vi "How to use in host.vi"(11 "Select Part":u16(ring) items=["P1.jpg", "P10.JPG", "P11.JPG", "P12.JPG", "P13.JPG", "P14.JPG", "P2.JPG", "P3.JPG", "P4.JPG", "P5.JPG", "P6.JPG", "P7.JPG", "P8.JPG", "P9.JPG"]) -> (1 "2D Picture":picture)   [LabVIEW 2015]
panel:
  out "error out":errorcluster
  out "empty?":bool
  in  "stop":bool
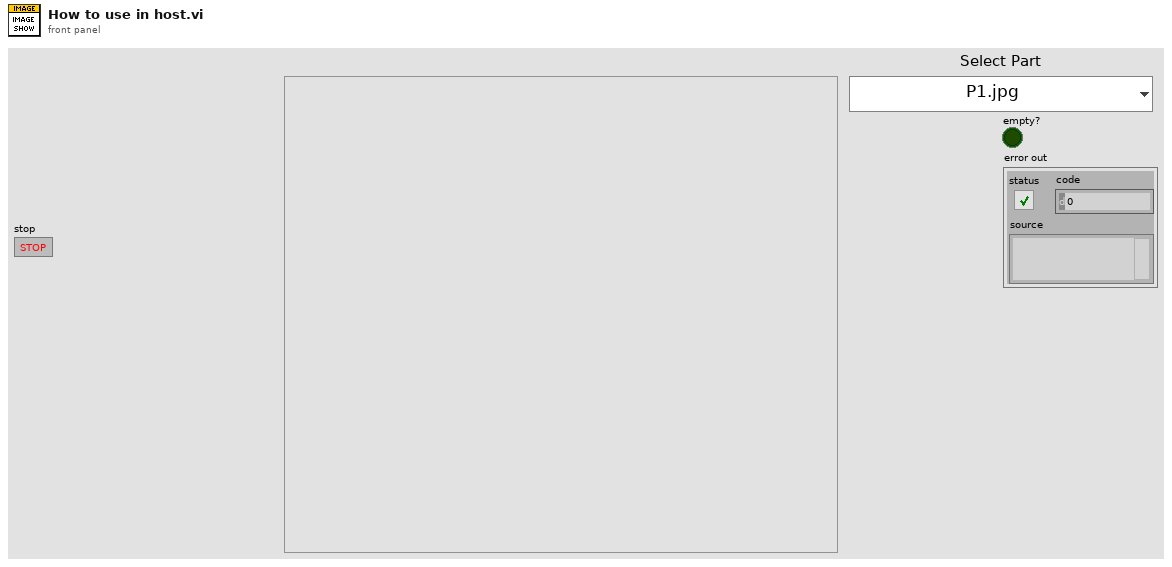
[diagram p1: front panel]
types:
  T1 = typedef "imagedata.ctl" = cluster{"image type":i32, "image depth":i32, "image":u8[], "mask":u8[], "colors":u32[], "Rectangle":cluster{"left":i16, "top":i16, "right":i16, "bottom":i16}}
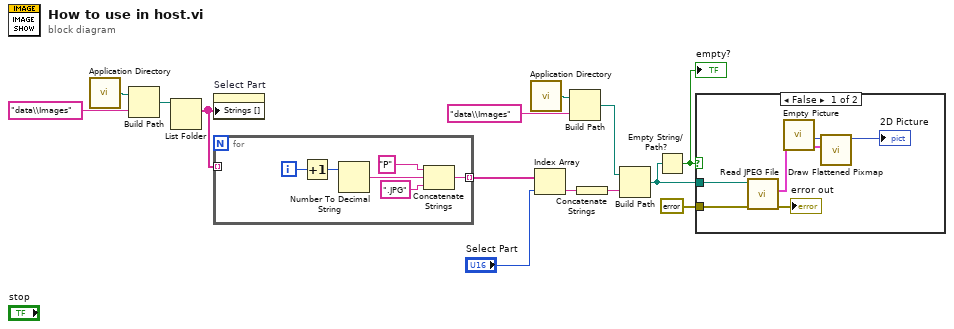
[diagram p0: block diagram]
diagram:
  n1 = call <vilib>:"Application Directory.vi"() -> ("Application Directory"=w14:path)
  n2 = Build Path(base path=w14, name or relative path="data\\Images") -> (appended path=w12:path)
  n3 = List Folder(path=w12) -> (filenames=w2:string[])  [unwired: 3 in, 3 out]
  n4 = property on="Select Part" class="Ring (strict)"("Strings []"=w2) -> ()  [unwired: 2 in, 2 out]
  n5 = for {
    tunnel: w2 -> [_] mode=indexing
    tunnel: [w15] -> w1 mode=indexing
    i -> [w19]
    n6 = Increment(x=w19) -> (x+1=w17:i32)
    n7 = Number To Decimal String(number=w17) -> (decimal integer string=w18:string)  [unwired: 1 in]
    n8 = Concatenate Strings("P" ("string"), w18, ".JPG" ("string")) -> (w15:string)
  }
  n9 = call <vilib>:"Application Directory.vi"() -> ("Application Directory"=w10:path)
  n10 = Index Array(array=w1, index="Select Part") -> (element=w7:string)
  n11 = Build Path(base path=w10, name or relative path="data\\Images") -> (appended path=w8:path)
  n12 = Concatenate Strings(w7) -> (w11:string)
  n13 = Build Path(base path=w8, name or relative path=w11) -> (appended path=w6:path)
  n14 = Empty String/Path?(string/path=w6) -> (empty?=w5:bool)
  "empty?" <- w5
  n15 = case shown="False" w5 {
    tunnel: w6 -> [w23 _]
    tunnel: errorcluster {"status"=FALSE, "code"=0, "source"=""} ("error in (no error)") -> [w22 _]
    frame False {
      n16 = call <vilib>:"Read JPEG File.vi"("error in (no error)"=w22, "path to JPEG file"=w23) -> ("error out"=→"error out":errorcluster, "image data"=w25:T1)  [unwired: 7 in, 1 out]
      n17 = call "Empty Picture"() -> ("empty picture"=w26:picture)
      n18 = call <vilib>:"Draw Flattened Pixmap.vi"("image data"=w25, "picture"=w26) -> ("new picture"=→"2D Picture":picture)  [unwired: 7 in]
    }
    frame True {
    }
  }
